vi "TemplateMethod.vi"(8 "ErrorIn":errorcluster, 9 "DummyIn":dbl, 11 "OpenCVCamIn":refnum<class "OpenCVCam.lvclass">) -> (0 "ErrorOut":errorcluster, 1 "DummyOut":dbl, 3 "OpenCVCamOut":refnum<class "OpenCVCam.lvclass">)   [LabVIEW 2021, in "OpenCVCam.lvclass"]
uses:
  OpenCVCam.lvclass
  C:/Localdata/Projects/TriekselSoft/TriekselsoftApplicationFramework/Source/.Externals/Library_YAF/YActor/YActor.lvclass
  Library_YAF/YActor/YActor.lvclass/YActor.ctl
  Library_YAF/YActor/ExeCmd_sync.vi
  Library_YAF/YActor/private/SendCommand.vi
  Library_YAF/YActor/private/WaitForReply.vi
  Library_YAF/YActor/private/CreateLocalVI.vi
  Library_YAF/YActor/private/ExeuteInlineVI.vi
  Library_YAF/YActor/private/GetRemoteVIRef.vi
  Library_YAF/YActor/private/GetNameOfVI.vi
  Library_YAF/YActor/QuickCast.vi
  Library_YAF/YActor/private/VINameProperty.vi
  Library_YAF/YActor/private/MessageCounter.vi
  Library_YAF/YActor/InlineReferencePool.vi
  Library_YAF/YActor/private/ExecuteVI.vi
  Library_YAF/YActor/YActor.lvclass
  C:/Localdata/Projects/TriekselSoft/TriekselsoftApplicationFramework/Source/.Externals/Library_YAF/YAFTAF/YAFTAF.lvclass
  C:/Localdata/Projects/TriekselSoft/TriekselsoftApplicationFramework/Source/.Externals/Interface_UserInterface_IFrontPanel/IFrontPanel/IFrontPanel.lvclass
  C:/Localdata/Projects/TriekselSoft/TriekselsoftApplicationFramework/Source/.Externals/Interface_TAF_IInterface/IInterface/IInterface.lvclass
  C:/Localdata/Projects/TriekselSoft/TriekselsoftApplicationFramework/Source/.Externals/Interface_Object_ICreateDestroy/ICreateDestroy/ICreateDestroy.lvclass
  C:/Localdata/Projects/TriekselSoft/TriekselsoftApplicationFramework/Source/.Externals/Interface_Object_IPersistentData/IPersistentData/IPersistentData.lvclass
  C:/Localdata/Projects/TriekselSoft/TriekselsoftApplicationFramework/Source/.Externals/Interface_TAF_ITAFObject/ITAFObject/ITAFObject.lvclass
  C:/Localdata/Projects/TriekselSoft/TriekselsoftApplicationFramework/Source/.Externals/YAFTAFModule_OpenCV_Camera/OpenCVCam/OpenCVCam.lvclass
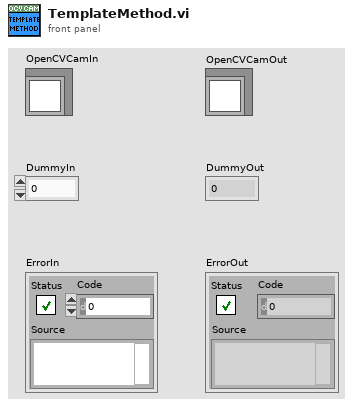
[diagram p1: front panel]
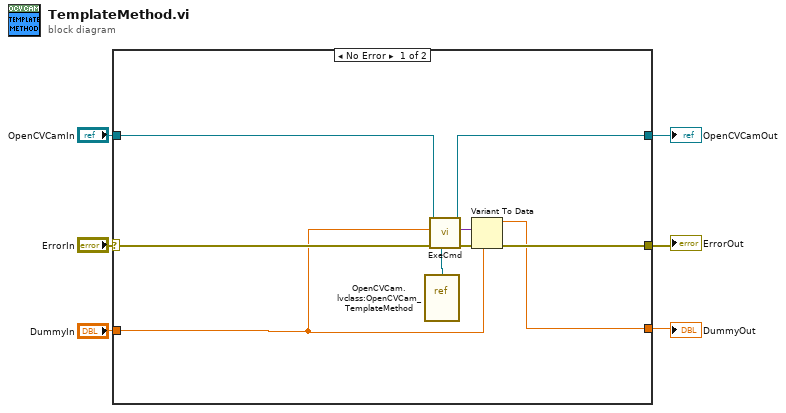
[diagram p0: block diagram]
diagram:
  n1 = case shown="No Error" "ErrorIn" {
    selector: "ErrorIn" -> [w15 w17]
    tunnel: [w13 w17] -> w5
    tunnel: [w9 w16] -> w3
    tunnel: "OpenCVCamIn" -> [w10 w16]
    tunnel: "DummyIn" -> [w8 _]
    tunnel: [w7 _] -> w1
    frame No Error {
      n2 = vi-ref "OpenCVCam.lvclass:OpenCVCam_TemplateMethod.vi"() -> (w12:refnum<vi>)
      n3 = call-poly "ExeCmd.vi"("CmdVIRef"=w12, "ErrorIn"=w15, "CmdData"=w8, "YActorIn"=w10) -> ("ErrorOut"=w14:errorcluster, "ReplyData"=w11:variant, "YActorOut"=w9:refnum<class "OpenCVCam.lvclass">)  [unwired: 5 in]
      n4 = Variant To Data(error in=w14, type=w8, Variant=w11) -> (data=w7:dbl, error out=w13:errorcluster)
    }
    frame Error {
    }
  }
  "ErrorOut" <- w5
  "OpenCVCamOut" <- w3
  "DummyOut" <- w1
